vi "PH_AWG-510.PSDB Trigger Settings.vi"(0 "i ref in":refnum<vi>, 5 "error IO":errorcluster) -> (14 "i ref out":refnum<vi>, 15 "Trigger Settings PSDB String Data":T2[](array[typedef]), 16 "Trigger Settings PSDB Numeric Data":T3[](array[typedef]), 18 "Trigger Settings PSDB Boolean Data":T4[](array[typedef]), 19 "error out":errorcluster)   [LabVIEW 2014, in "PH_AWG-510.lvlib"]
doc: "This VI sets the data of the output settings for the PSDB."
uses:
  PH_AWG-510.lvlib
  PH_Basics/PH_PSDBWriter/PH_PSDBWriter.Boolean dataset.ctl
  PH_Basics/PH_PSDBWriter/PH_PSDBWriter.Numeric dataset.ctl
  PH_Basics/PH_PSDBWriter/PH_PSDBWriter.String dataset.ctl
  PH_Basics/PH_PSDBWriter/PH_PSDBWriter.lvlib
panel:
  in  "Current Settings.Trigger.Mode":T1(ring)
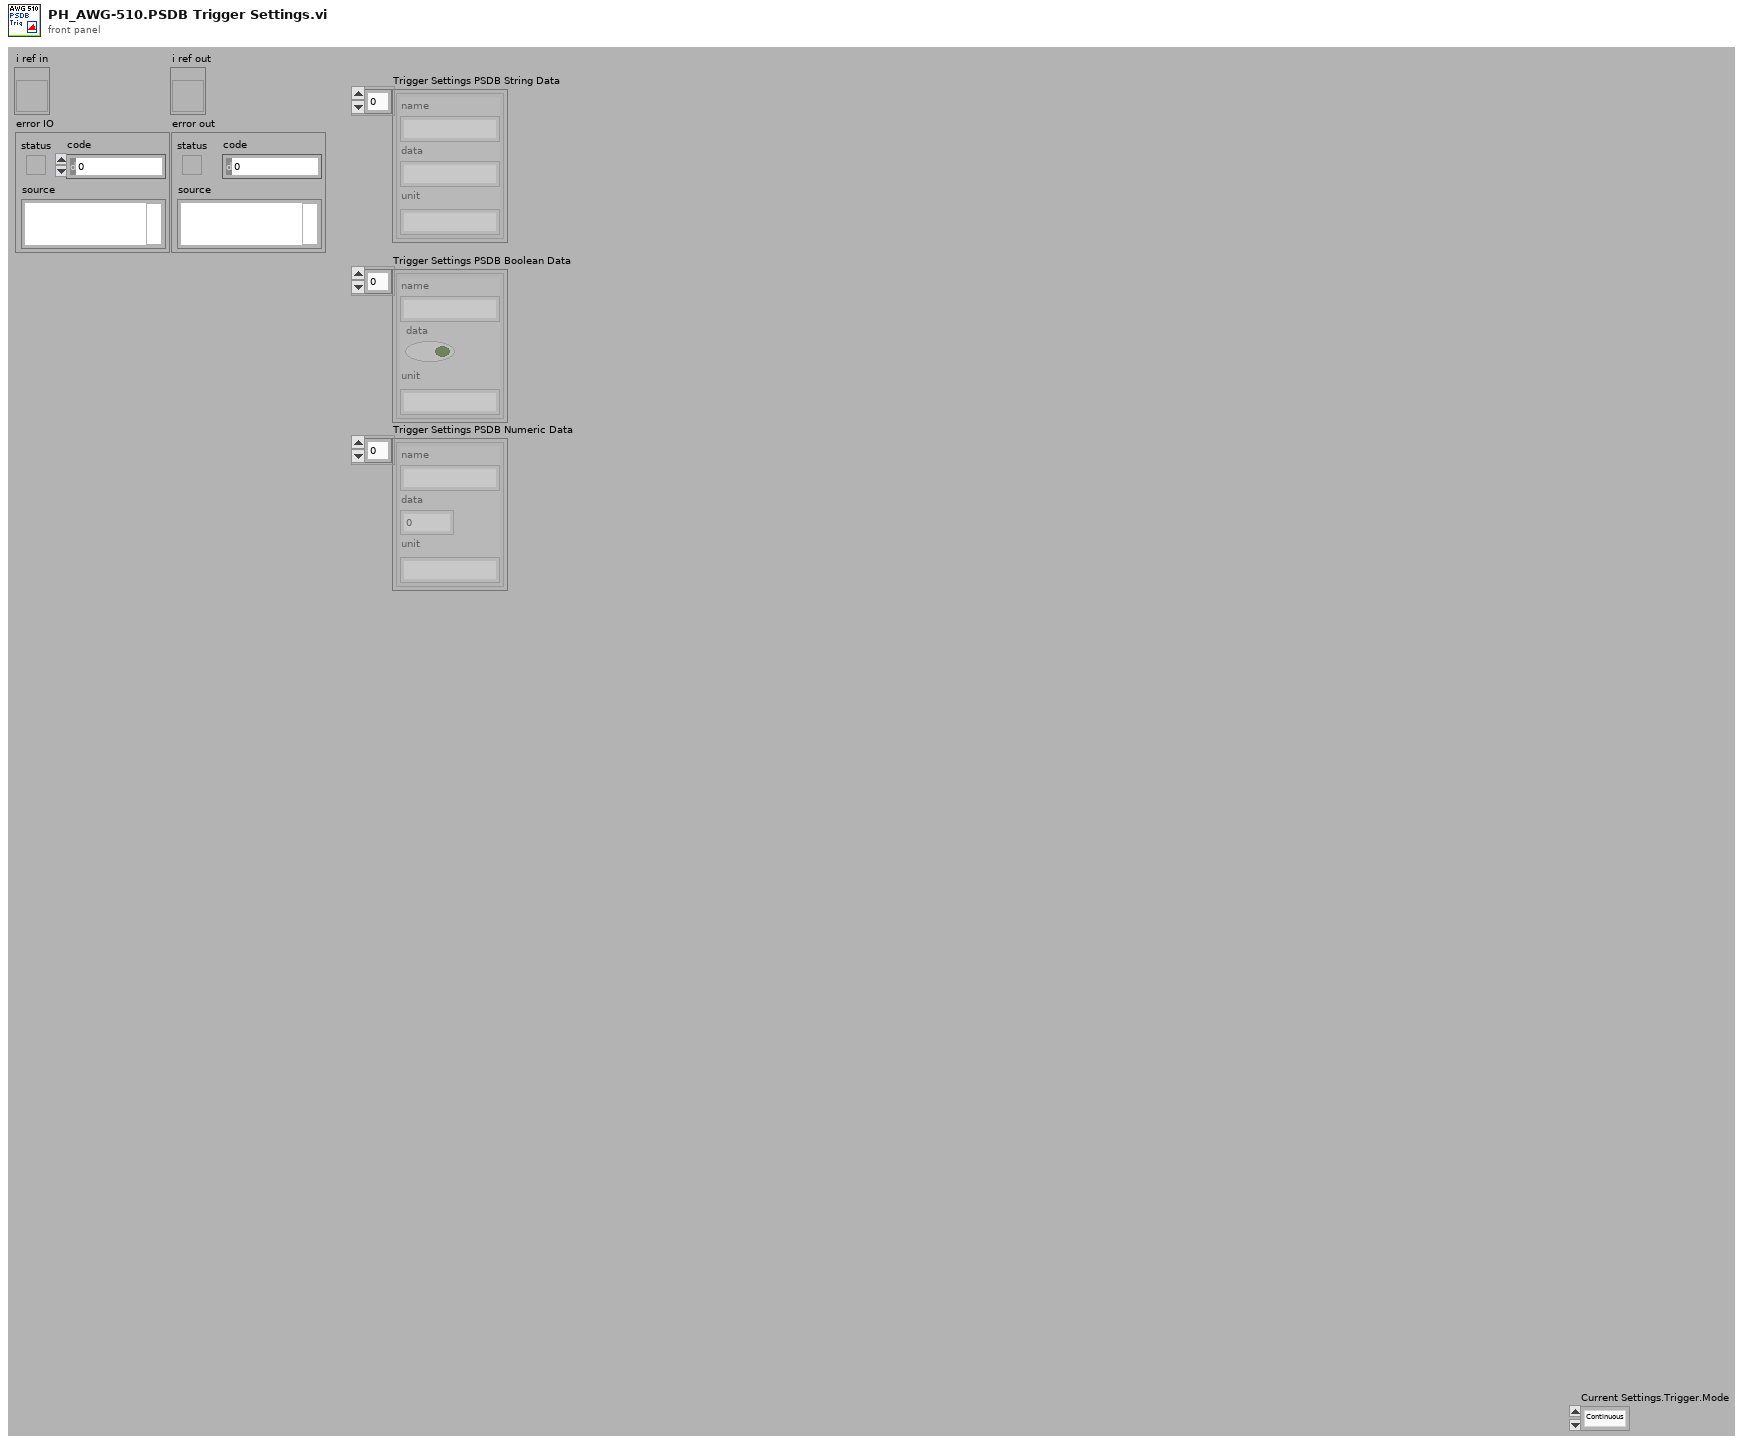
[diagram p1: front panel]
types:
  T1 = enum16{"Continuous", "Triggered", "Gated", "Enhanced"}
  T2 = typedef "PH_PSDBWriter.lvlib/PH_PSDBWriter.String dataset.ctl" = cluster{"name":string, "data":string, "unit":string}
  T3 = typedef "PH_PSDBWriter.lvlib/PH_PSDBWriter.Numeric dataset.ctl" = cluster{"name":string, "data":dbl, "unit":string}
  T4 = typedef "PH_PSDBWriter.lvlib/PH_PSDBWriter.Boolean dataset.ctl" = cluster{"name":string, "data":bool, "unit":string}
  T5 = typedef "PH_AWG-510.lvlib/PH_AWG-510.i attribute.ctl" = cluster{"GUI Refs":cluster{"Delete":refnum<vi>, "Trigger Settings":refnum<vi>, "Start Device":refnum<vi>, "Instrument Information":refnum<vi>, "Lock Frontpanel":refnum<vi>, "Waveform Pattern File":refnum<vi>, "Initialize":refnum<vi>, "Output Settings":refnum<vi>}, "Instrument Information":T6, "Initialized?":bool, "Current Settings":cluster{"Trigger":T7, "Output Settings":T8}, "Wanted Settings":cluster{"Trigger":T7, "Output Settings":T8}, "Device frontpanel locked?":bool, "Default File Path":path}
  T6 = typedef "PH_AWG-510.lvlib/PH_AWG-510.Instrument Information Dataset.ctl" = cluster{"VISA resource name":refnum<visa-resource-name>, "Instrument Firmware Revision":string, "Manufacturer":string, "Model":string, "Serial Number":string, "Error Message":string, "Device Status":enum16{"stopped", "wating for trigger", "running", "Failure"}}
  T7 = typedef "PH_AWG-510.lvlib/PH_AWG-510.Trigger Settings.ctl" = cluster{"Mode":enum16{"Continuous", "Triggered", "Gated", "Enhanced"}, "Level (V)":dbl, "External Source":bool}
  T8 = typedef "PH_AWG-510.lvlib/PH_AWG-510.Output Settings.ctl" = cluster{"Activate Channel":bool, "VPP (V)":dbl, "Clock (Hz)":dbl, "File Name (Device)":string, "#1":u16, "#2":u16, "#3":u16, "#4":u16, "#5":u16, "#6":u16, "#7":u16, "#8":u16, "#9":u16, "#10":u16, "#11":u16, "#12":u16, "#13":u16, "#14":u16, "#15":u16, "#16":u16, "#17":u16, "#18":u16, "#19":u16, "#20":u16, "Offset (V)":dbl}
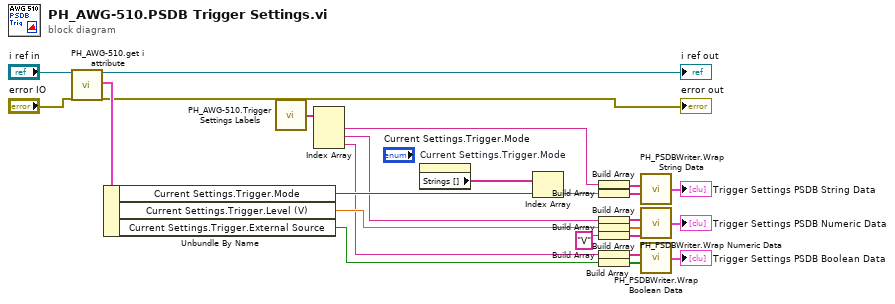
[diagram p0: block diagram]
diagram:
  n1 = call "PH_AWG-510.get i attribute.vi"("i ref in"="i ref in", "error in (no error)"="error IO") -> ("i ref out"=→"i ref out":refnum<vi>, "i attribute"=w23:T5, "error out"=→"error out":errorcluster)  [unwired: 15 in]
  n2 = Unbundle By Name(w23) -> ("Current Settings.Trigger.Mode"=w11:T1, "Current Settings.Trigger.Level (V)"=w3:dbl, "Current Settings.Trigger.External Source"=w1:bool)
  n3 = call "PH_AWG-510.Trigger Settings Labels.vi"() -> ("Trigger Settings Labels"=w19:string[])
  n4 = Index Array(array=w19) -> (element #1=w9:string, element #2=w4:string, element #3=w2:string)  [unwired: 3 in]
  n5 = property on="Current Settings.Trigger.Mode" class="Enum (strict)"() -> ("Strings []"=w12:string[])  [unwired: 2 in, 2 out]
  n6 = Index Array(array=w12, index=w11) -> (element=w10:string)
  n7 = Build Array(w9) -> (w17:string[])
  n8 = Build Array(w10) -> (w22:string[])
  n9 = Build Array(w4) -> (w5:string[])
  n10 = Build Array(w3) -> (w6:dbl[])
  n11 = Build Array("V") -> (w7:string[])
  n12 = Build Array(w2) -> (w18:string[])
  n13 = Build Array(w1) -> (w20:bool[])
  n14 = call "PH_PSDBWriter.Wrap String Data.vi"("Data Array"=w22, "Name Array"=w17) -> ("PSDB String Data Array"=→"Trigger Settings PSDB String Data":T2[])  [unwired: 2 in]
  n15 = call "PH_PSDBWriter.Wrap Numeric Data.vi"("Unit Array"=w7, "Data Array"=w6, "Name Array"=w5) -> ("PSDB Numeric Data Array"=→"Trigger Settings PSDB Numeric Data":T3[])  [unwired: 1 in]
  n16 = call "PH_PSDBWriter.Wrap Boolean Data.vi"("Data Array"=w20, "Name Array"=w18) -> ("PSDB Boolean Data Array"=→"Trigger Settings PSDB Boolean Data":T4[])  [unwired: 2 in]
